vi "4.6.3.vi"(0 "停止":bool, 2 "数值 2":dbl, 3 "数值":dbl) -> (1 "x+y":dbl)   [LabVIEW 2017]
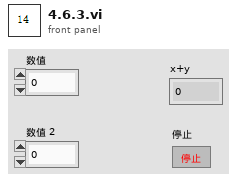
[diagram p1: front panel]
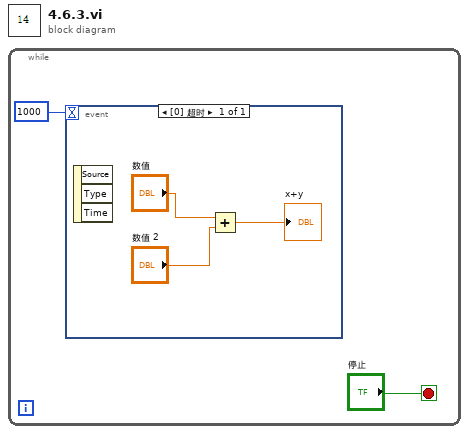
[diagram p0: block diagram]
diagram:
  n1 = while {
    stop <- "停止" stop-if-true
    n2 = event shown="[0] 超时" {
      selector: _ -> [_]
      dyn-events: _ -> [_]
      timeout: 1000 -> [_]
      event Timeout {
        n3 = event-data() -> ()  [unwired: 1 in, 3 out]
        n4 = Add(x="数值", y="数值 2") -> (x+y=→"x+y":dbl)
      }
    }
  }
